vi "Configure Session.vi"(8 "error in (no error)":errorcluster, 11 "RandomNumberGenerator in":refnum<class "RandomNumberGenerator.lvclass">) -> (0 "error out":errorcluster, 3 "RandomNumberGenerator out":refnum<class "RandomNumberGenerator.lvclass">)   [LabVIEW 2020, in "RandomNumberGenerator.lvlib" / "RandomNumberGenerator.lvclass"]
doc: "<b>Configure Session</b>\nCalled once per session, and is always called after the plugin loads its configuration\n\nFor the ADAS use case, we typically only have a single session of a plugin during a run. In the future we may add the ability to support multiple sessions.\n\nIn this VI, take the configuration parameters and call the appropriate initialization functions to open and store any references needed during the run. For example, call Open/Create/Replace File on the path stored in configuration and store the file reference as part of the class private data for the plugin class.\n\nIf your plugin needs information from the configuration to decide what timing parameters to use (for example, to configure the period of a Periodic timing), set those here instead of in the Initialize function."
uses:
  RandomNumberGenerator.lvclass
  RandomNumberGenerator.lvclass/RandomNumberGenerator.ctl
  <vilib>/ADAS Record/Utilities/ADAS Utilities.lvlib
  <vilib>/FlexLogger/SDK/PluginSDK.lvlibp/PEFClasses/SDK/Processing Element/Processing Element.lvclass
  <vilib>/FlexLogger/SDK/PluginSDK.lvlibp/PEFClasses/SDK/Processing Element/Timing Method.ctl
  <vilib>/FlexLogger/SDK/PluginSDK.lvlibp/PEFClasses/SDK/Processing Element/Timing Parameters.ctl
  C:/Program Files/National Instruments/LabVIEW 2020/vi.lib/FlexLogger/SDK/PluginSDK.lvlibp/PEFClasses/SDK/Processing Element/Processing Element.lvclass
  C:/Projects/GitHub/data-record-ad/IO Plugins/RandomNumberGenerator/PE/RandomNumberGenerator.lvclass
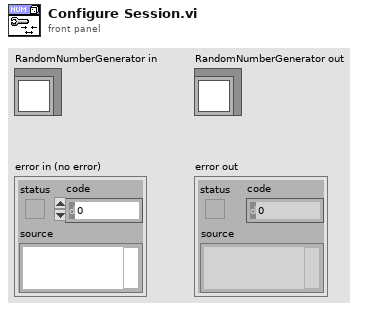
[diagram p1: front panel]
types:
  T1 = typedef "PluginSDK.lvlibp/Processing Element.lvclass/Timing Parameters.ctl" = cluster{"Timing Method":T2, "Timing Period (ms)":i32}
  T2 = typedef "PluginSDK.lvlibp/Processing Element.lvclass/Timing Method.ctl" = enum16{"Periodic", "Immediate", "On Data Ready", "Triggered"}
  T3 = typedef "RandomNumberGenerator.lvlib/RandomNumberGenerator.lvclass/Configuration.ctl" = cluster{"Lower Bound":dbl, "Upper Bound":dbl, "# Elements":i32, "Update Rate (ms)":i32}
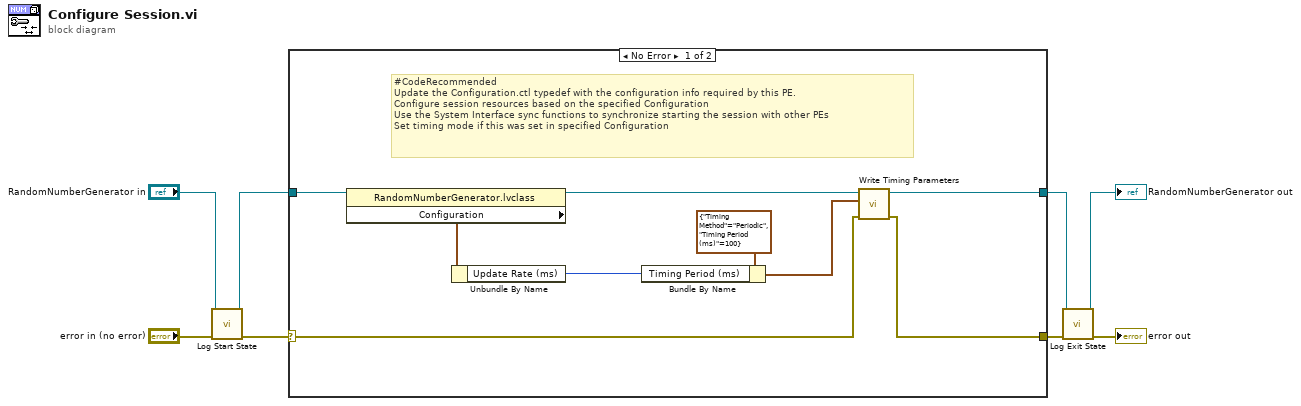
[diagram p0: block diagram]
diagram:
  n1 = call <vilib>:"Log Start State.vi"("error in (no error)"="error in (no error)", "PluginSDK.lvlibp:Processing Element.lvclass"="RandomNumberGenerator in") -> ("error out"=w7:errorcluster, "PluginSDK.lvlibp:Processing Element.lvclass"=w5:refnum<class "RandomNumberGenerator.lvclass">)  [unwired: 8 in]
  n2 = case shown="No Error" w7 {
    selector: w7 -> [w12 w18]
    tunnel: w5 -> [w17 w19]
    tunnel: [w13 w19] -> w2
    tunnel: [w11 w18] -> w4
    frame No Error {
      # "#CodeRecommended\nUpdate the Configuration.ctl typedef with the configuration info required by this PE.\nConfigure session resources based on the specified Configuration\nUse the System Interface sync functions to synchronize starting the session with other PEs\nSet timing mode if this was set in specified Configuration"
      n3 = property on="Property Node" class="RandomNumberGenerator.lvclass"(reference=w17) -> (reference out=w14:refnum<class "RandomNumberGenerator.lvclass">, "Configuration"=w15:T3)  [unwired: 1 in, 1 out]
      n4 = Unbundle By Name(w15) -> ("Update Rate (ms)"=w10:i32)
      n5 = Bundle By Name(cluster=T1 {"Timing Method"=enum."Periodic", "Timing Period (ms)"=100} ("Timing Parameters"), "Timing Period (ms)"=w10) -> (w9:T1)
      n6 = call <vilib>:"Write Timing Parameters.vi"("error in (no error)"=w12, "Timing Parameters"=w9, "PEF Processing Element in"=w14) -> ("error out"=w11:errorcluster, "PEF Processing Element out"=w13:refnum<class "RandomNumberGenerator.lvclass">)  [unwired: 7 in]
    }
    frame Error {
    }
  }
  n7 = call <vilib>:"Log Exit State.vi"("error in (no error)"=w4, "PluginSDK.lvlibp:Processing Element.lvclass"=w2) -> ("error out"=→"error out":errorcluster, "PluginSDK.lvlibp:Processing Element.lvclass"=→"RandomNumberGenerator out":refnum<class "RandomNumberGenerator.lvclass">)  [unwired: 8 in]
